vi "Avery Tronix StandAlone.vi"(8 "Error In":errorcluster) -> (0 "Error Out":errorcluster)   [LabVIEW 2016]
uses:
  <vilib>/NI/Modbus Library/API/Wrapper/Create TCP Master.vi
  <vilib>/NI/Modbus Library/API/Master/Modbus Master.lvclass
  <vilib>/NI/Modbus Library/API/Wrapper/API Main.lvlib
panel:
  in  "Remote IP Address":string="10.0.3.5"
  in  "stop":bool
  out "Avery Weigth Tronix Data":string[](array[string])=["Weight (Lbs)", "29.800"]
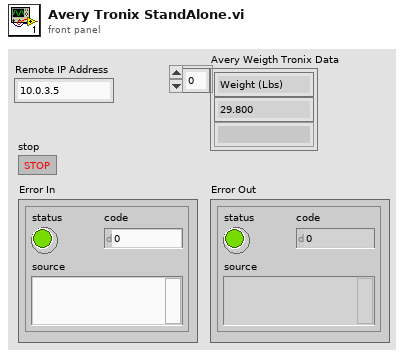
[diagram p1: front panel]
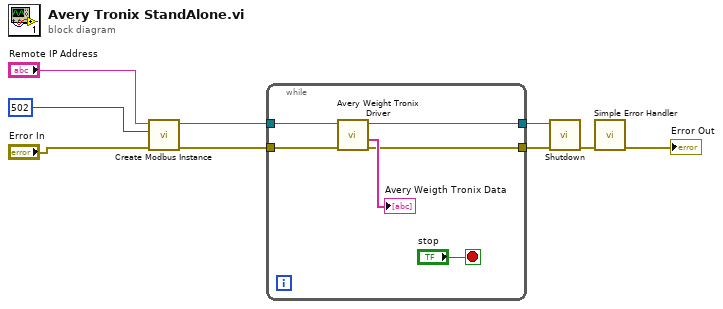
[diagram p0: block diagram]
diagram:
  n1 = call-poly <vilib>:"Create Modbus Instance.vi"("error in"="Error In", "port (502)"=u16 502 ("Remote Port"), "address"="Remote IP Address") -> ("error out"=w2:errorcluster, "TCP master instance"=w3:refnum<class "Modbus Master.lvclass">)  [unwired: 7 in]
  n2 = while {
    tunnel: [w13] -> w7
    tunnel: [w12] -> w6
    tunnel: w3 -> [w11]
    tunnel: w2 -> [w10]
    stop <- "stop" stop-if-true
    n3 = call "Avery Weight Tronix Driver.vi"("error in (no error)"=w10, "Modbus master in"=w11) -> ("error out"=w13:errorcluster, "Avery Weigth Tronix Data"=→"Avery Weigth Tronix Data":string[], "Modbus master out"=w12:refnum<class "Modbus Master.lvclass">)  [unwired: 6 in, 1 out]
  }
  n4 = call-dynamic "Shutdown.vi"("error in"=w7, "Modbus master in"=w6) -> ("error out"=w9:errorcluster)  [unwired: 9 in]
  n5 = call <vilib>:"Simple Error Handler.vi"("error in (no error)"=w9) -> ("error out"=→"Error Out":errorcluster)  [unwired: 1 in, 7 out]
